vi "Configure Fold-Back Protection.vi"(7 "Slave Address":i32=-1 min=-1 max=30 step=1, 8 "error":errorcluster, 10 "Fold-Back ON":bool, 11 "VISA":refnum<visa-resource-name>) -> (0 "error out":errorcluster, 3 "VISA out":refnum<visa-resource-name>)   [LabVIEW 2025, in "TDK-Lambda GEN LAN Series.lvlib"]
doc: "Configure the Fold-Back (or over-current) protection ON or OFF. The FB protection is tripped when the power supply goes into Constant-Current mode (as if the load goes into a short-circuit)\n\nNote: After a FB shutdown, the output can be turned ON by running the \"Configure Output On-Off.vi\" driver"
uses:
  <userlib>/TDK-Lambda GEN LAN Series/TDK-Lambda GEN LAN Series.lvlib
panel:
  # "TDK-Lambda Genesys \n LAN\n  DC Power Supplies"
  # "Set Fold-Back \nProtection (FB) \nON or OFF"
  # "(c) 2019 TDK-Lambda.  ALL RIGHTS RESERVED."
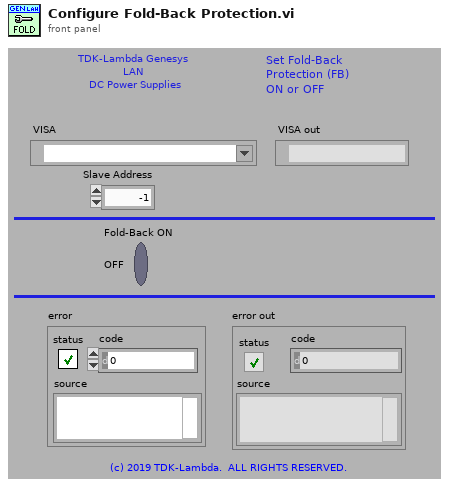
[diagram p1: front panel]
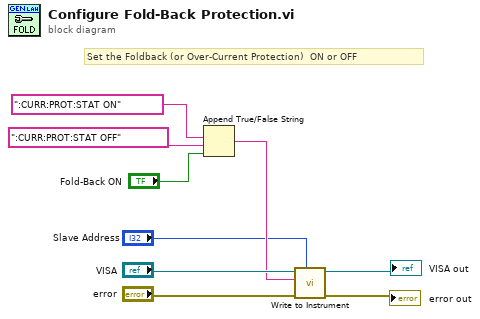
[diagram p0: block diagram]
diagram:
  # "Set the Foldback (or Over-Current Protection)  ON or OFF"
  n1 = Append True/False String(1:"Fold-Back ON", 2:":CURR:PROT:STAT OFF" ("format string"), 3:":CURR:PROT:STAT ON" ("format string")) -> (0:w4:string)  [unwired: 1 in]
  n2 = call <userlib>:"Write to Instrument.vi"("Slave Address"="Slave Address", "error"="error", "Command"=w4, "VISA"="VISA") -> ("error out"=→"error out":errorcluster, "VISA out"=→"VISA out":refnum<visa-resource-name>)  [unwired: 6 in]
